vi "Fpga-MicroBlaze_lwIP.vi"() -> ()   [LabVIEW 2017, in "My Network FPGA v1.lvlib"]
uses:
  Example SubVIs/My Network FPGA v1.lvlib
  <instrlib>/_niInstr/Streaming/v1/Common/Stream State.ctl
  <vilib>/Platform/TimedLoop/XDataNode/timing_clust.ctl
  <vilib>/Platform/TimedLoop/XDataNode/nitl_modes.ctl
  <vilib>/Platform/TimedLoop/XDataNode/wakeup.ctl
  <instrlib>/_niInstr/Network/Ethernet/MAC/CLIP/v1/Resources.ctl
  Example SubVIs/TX Controls.ctl
  <instrlib>/_niInstr/Network/Ethernet/MAC/CLIP/v1/niInstr Ethernet MAC - CLIP v1.lvclass
  C:/Program Files (x86)/National Instruments/LabVIEW 2017/instr.lib/_niInstr/Network/Ethernet/MAC/API/v1/FPGA/niInstr Ethernet MAC v1.lvclass
  <instrlib>/_niInstr/Network/API/v1/FPGA/Address Space/niInstr Network API FPGA Address Space v1.lvclass
  C:/Program Files (x86)/National Instruments/LabVIEW 2017/instr.lib/_niInstr/Instruction Framework/v1/FPGA/Interfaces/Address Space Collection/Address Space Collection.lvclass
  <instrlib>/_niInstr/FIFO Register Bus/v1/FPGA/niInstr FIFO Register Bus v1 FPGA.lvclass
  C:/Program Files (x86)/National Instruments/LabVIEW 2017/instr.lib/_niInstr/Instruction Framework/v1/FPGA/Interfaces/Instruction Producer/Instruction Producer.lvclass
  <vilib>/rvi/Emulation/niFpgaSctlEmulationGetInTimedLoop.vi
  <vilib>/rvi/Emulation/niFpgaEmulationReportErrorSimple.vi
  <vilib>/rvi/Emulation/niFpgaGetClockAttributes.vi
  <vilib>/rvi/Emulation/niFpgaCriticalErrorInLSC.vi
  <vilib>/rvi/eio/common/nirviEmuTemplateMethod_errors.vi
  <vilib>/rvi/interface/RandomDataEmulation/niFpgaRandomDataHandleErrors.vi
  <vilib>/Platform/TimedLoop/XDataNode/XDataNode.xnode
  <vilib>/eio/EIONode/EIONode.xnode
  <vilib>/rvi/DataTransferAndStorage/Container/XNode/niFpgaContainer.xnode
  <vilib>/rvi/interface/RandomDataEmulation/nirviRandomDataFpgaReadWriteTemplate.vi
  <vilib>/Platform/TimedLoop/XDataNode/XDNodeRunTimeDep.lvlib
  <instrlib>/_niInstr/Instruction Framework/v1/FPGA/Top Level Bus/Register Configuration/Register Configuration.lvclass
  <instrlib>/_niInstr/Network/API/v1/FPGA/niInstr Network API FPGA v1.lvclass
  <instrlib>/_niInstr/Streaming/v1/Common/niInstr Streaming v1 Common.lvlib
panel:
  out "AXI_STR_RXD_tready 1":bool
  out "tvalid 1":bool
  out "tdata 1":u32
  out "tlast 1":bool
  out "AXI_STR_RXD_tready_Count 1":u16
  out "tvalid_Count 1":u16
  out "tlast_Count 1":u16
  out "tdata_LastNonZero 1":u32
  out "AXI_STR_RXD_tready 2":bool
  out "tvalid 2":bool
  out "tdata 2":u32
  out "tlast 2":bool
  out "AXI_STR_RXD_tready_Count 2":u16
  out "tvalid_Count 2":u16
  out "tlast_Count 2":u16
  out "tdata_LastNonZero 2":u32
  in  "GPIO #1 in":u32
  out "GPIO #1 out":u32
  in  "GPIO #2 in":u32
  out "GPIO #2 out":u32
  in  "Interrupt #0":bool
  in  "Interrupt #1":bool
  in  "Tab Control":T1(tab)
  in  "UDP Source Port 0":u16=43981
  in  "UDP Destination Port 0":u16=61185
  in  "preferred datagram size 0":u16=1472
  in  "Port 0 RX/TX":enum32{"RX", "TX"}(tab)
  in  "Port 0 RX Clear Counts":bool
  out "Port 0 RX Good Frames Count":u32
  out "Port 0 RX Error Frames Count":u32
  out "Port 0 RX Received Columns Count":u32
  out "Port 0 RX Dropped Columns Count":u32
  out "Port 0 RX Data":u64 format="%.0x"
  in  "stream.num samples 0":u64
  in  "stream.request state 0":T2
  out "stream.metadata 0":u64
  out "stream.samples transferred 0":u64
  out "stream.state 0":T2
  in  "Port 1 RX/TX":enum32{"RX", "TX"}(tab)
  in  "Use Pattern Gen":bool
  in  "max frame payload":u16=1472
  in  "minimum packet interval":u32=1
  out "mgtrefclks_locked":bool
  out "mgtrefclks_valid":bool
  out "posc_complete":bool
  out "aBlockLockPort0":bool
  out "aBlockLockPort1":bool
  out "sPort0_Power_Good":bool
  out "sPort1_Power_Good":bool
  out "signal_detect_Port0":bool
  out "signal_detect_Port1":bool
  in  "fifo reg bus ctrl 0":u32
  out "fifo reg bus status 0":u32
  out "fifo reg bus data 0":u64
  # "License Note\n\nThis example makes use of code under the LGPLv2 license in the Socketed CLIP to support 10 Gigabit Ethernet.  You may find the source and build instructions for this component in the CLIP directory."
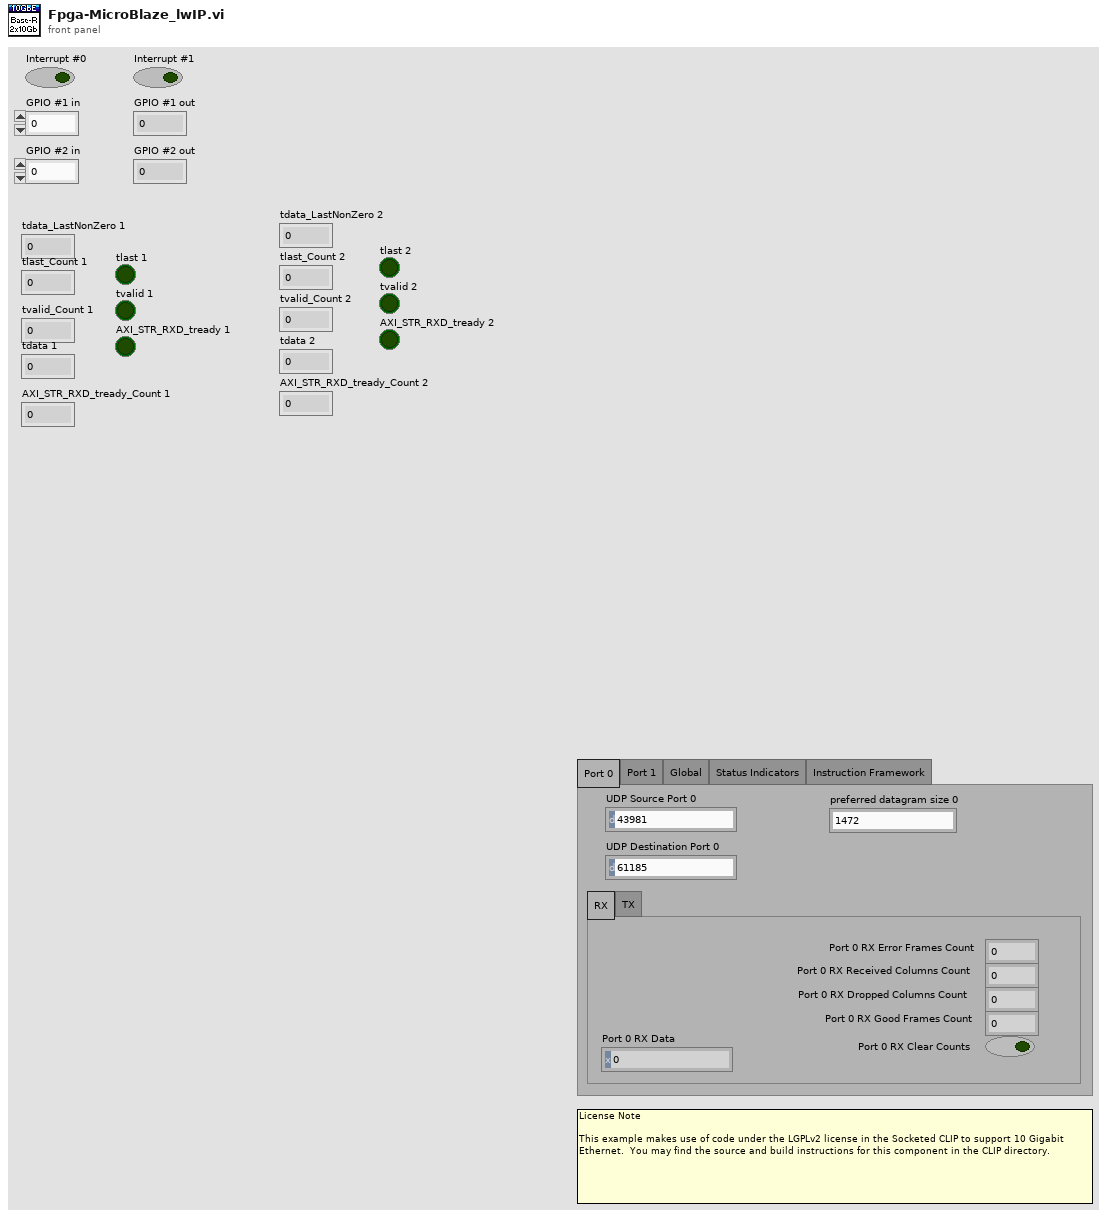
[diagram p1: front panel]
types:
  T1 = enum32{"Port 0", "Port 1", "Global", "Status Indicators", "Instruction Framework"}
  T2 = typedef "niInstr Streaming v1 Common.lvlib/Stream State.ctl" = enum8{"Idle", "Finite Transfer", "Continuous", "Done", "Error", "Not Ready", "Cancel"}
  T3 = typedef "niInstr Ethernet MAC - CLIP v1.lvclass/Resources.ctl" = cluster{"RX":cluster{"TData":refnum<k21>, "TValid":refnum<k21>, "TKeep":refnum<k21>, "TLast":refnum<k21>, "TUser":refnum<k21>}, "TX":cluster{"TData":refnum<k21>, "TValid":refnum<k21>, "TKeep":refnum<k21>, "TLast":refnum<k21>, "TReady":refnum<k21>}, "Pause resources":cluster{"cPauseValuePort":refnum<k21>, "cPauseReqPort":refnum<k21>}, "MAC Clock":refnum<k21>}
  T4 = typedef "XDNodeRunTimeDep.lvlib/timing_clust.ctl" = cluster{"Expected End [f-1]":u64, "Actual End [f-1]":u64, "Finished Late? [f-1]":bool, "Expected End [i-1]":u64, "Actual End [i-1]":u64, "Finished Late? [i-1]":bool, "Expected Start [i]":u64, "Actual Start [i]":u64, "Expected Start [f]":u64, "Actual Start [f]":u64, "Source Name":string, "Structure Name":string, "Period":i64, "Deadline":i64, "Offset":i64, "Start":i64, "Priority":i32, "Timeout":i32, "Mode":T5, "Wakeup Reason":T6, "Error":errorcluster, "Source Type":string, "Secondary Source Type":string, "Global End Time":u64, "Global Start Time":u64, "Frame Duration":u64, "Iteration Duration":u64, "Assigned CPU":i32, "I/O Scan Engine Mode":u32}
  T5 = typedef "XDNodeRunTimeDep.lvlib/nitl_modes.ctl" = enum32{"No Change", "Process missed periods, maintain original phase", "Discard missed periods, maintain original phase", "Process missed periods, ignore original phase", "Discard missed periods, ignore original phase"}
  T6 = typedef "XDNodeRunTimeDep.lvlib/wakeup.ctl" = enum32{"Normal", "Aborted", "Asynchronous wakeup", "Timing source error", "Timed loop error", "Timeout"}
  T7 = typedef "My Network FPGA v1.lvlib/TX Controls.ctl" = cluster{"UDP Source Port":u16, "UDP Destination Port":u16, "preferred datagram size":u16, "Use Pattern Gen":bool, "max frame payload":u16, "minimum packet interval":u32, "stream.num samples 0":u64, "stream.request state 0":T2}
  T8 = cluster{"Port RX Good Frames Count":u32, "Port RX Received Columns Count":u32, "Port RX Dropped Columns Count":u32, "Port RX Error Frames Count":u32, "Port RX Data":u64}
  T9 = typedef "My Network FPGA v1.lvlib/TX Indicators.ctl" = cluster{"stream.state 0":T2, "stream.metadata 0":u64, "stream.samples transferred 0":u64}
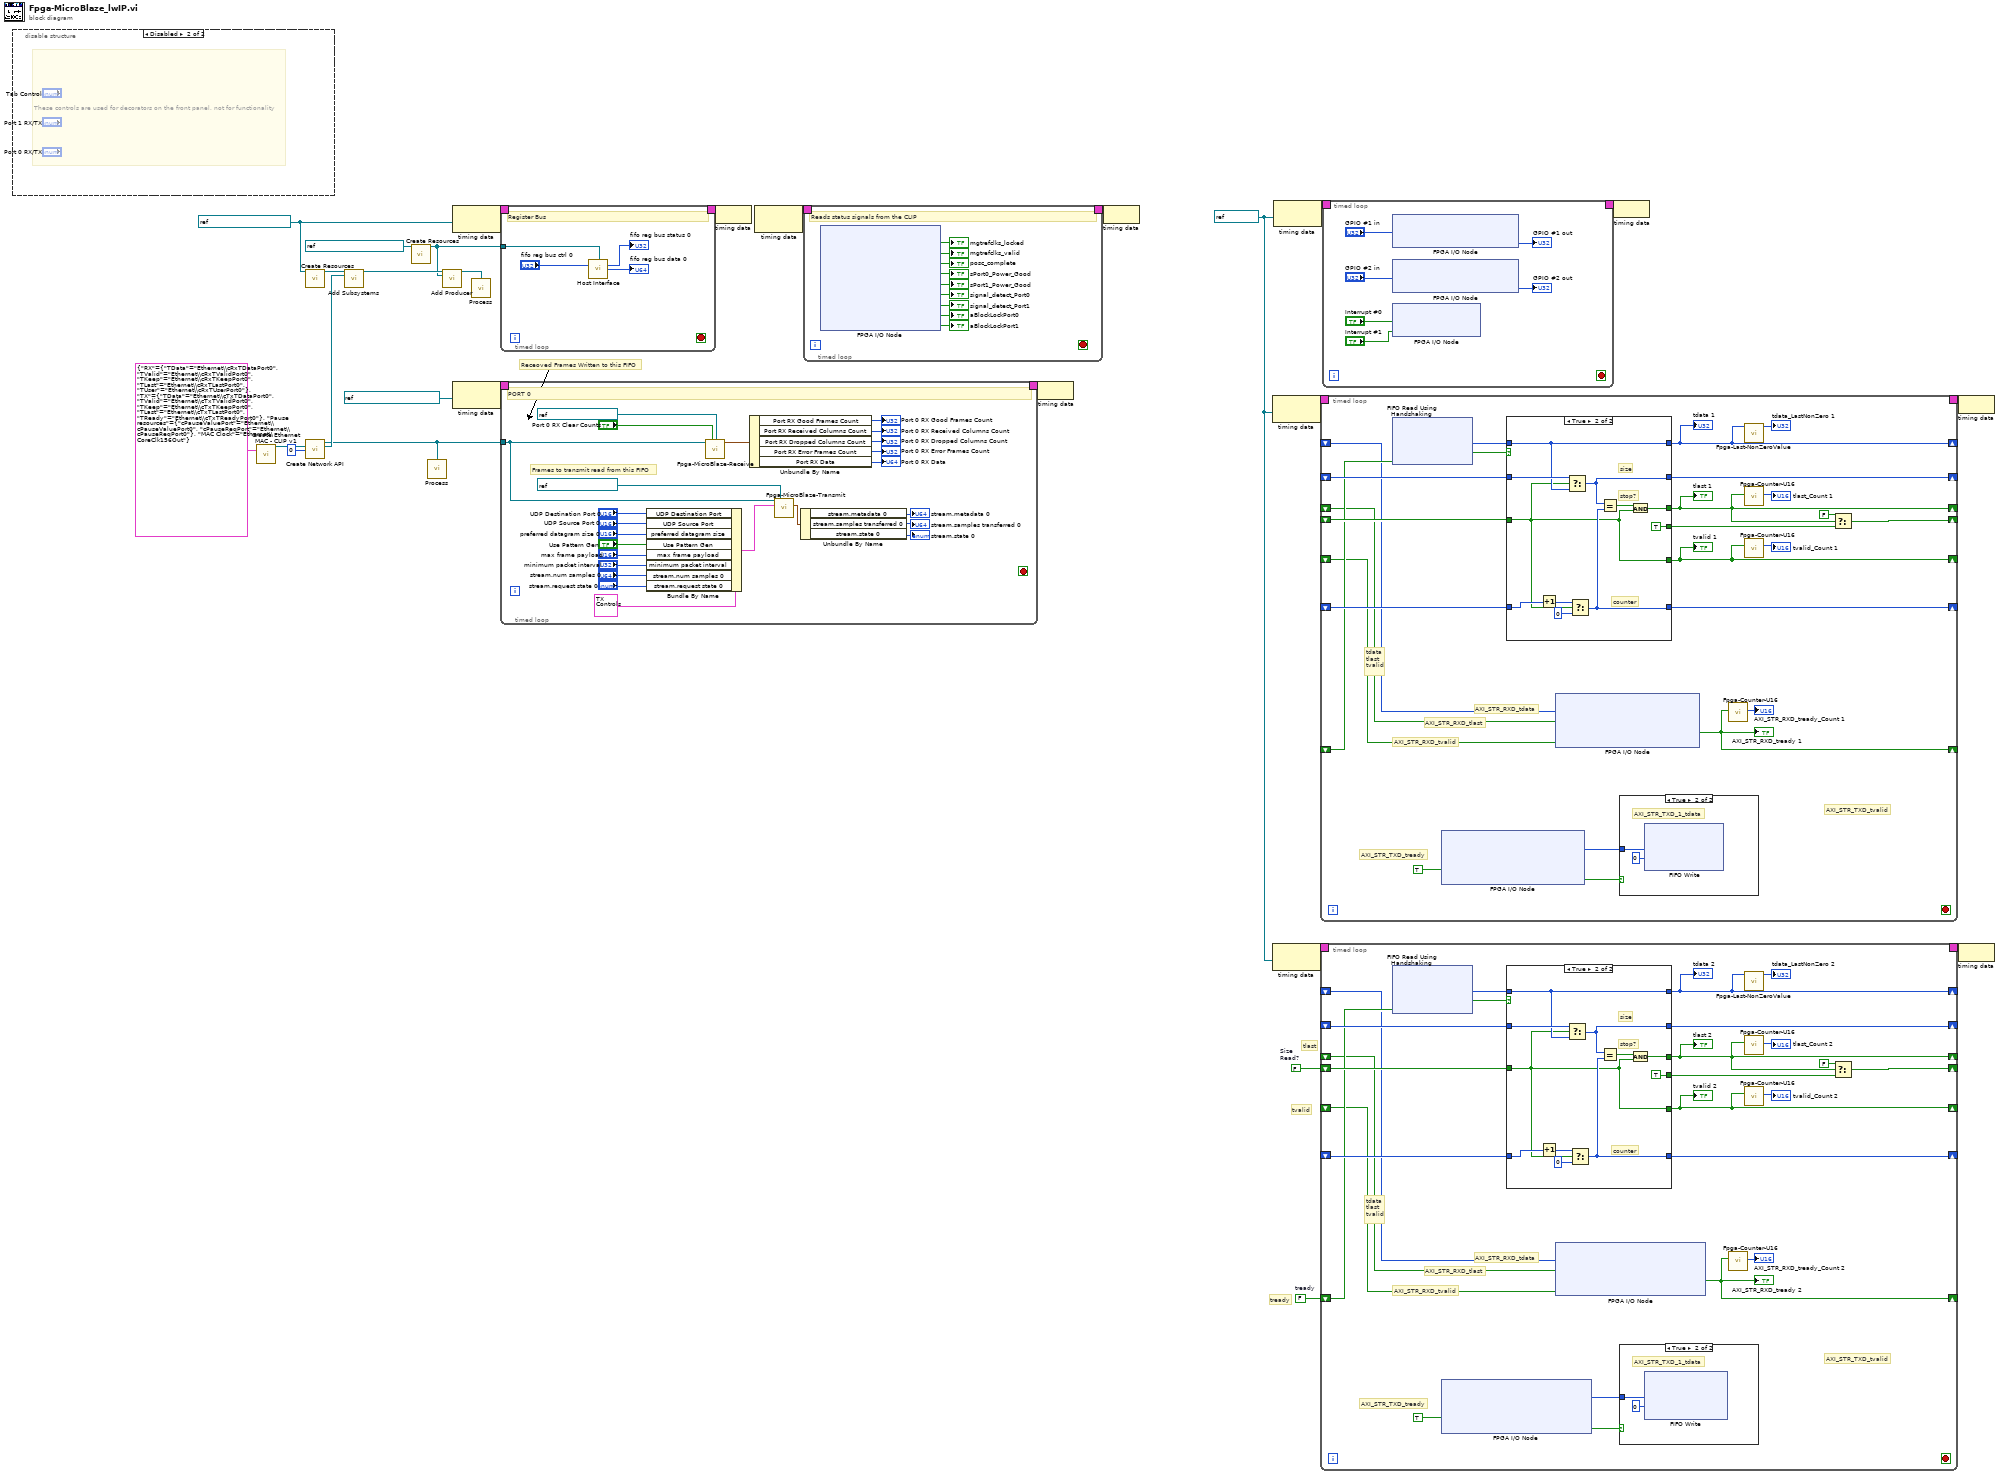
[diagram p0: block diagram]
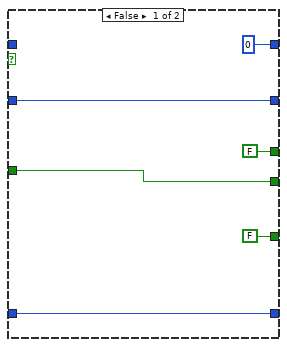
[diagram p3: hidden frame]
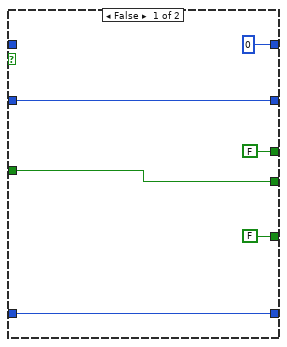
[diagram p5: hidden frame]
diagram:
  w2 = FALSE  # Size Read?
  w3 = FALSE  # tready
  w1 = refnum<k21> "100MHz" ("Source Name")
  w22 = refnum<k21> "40 MHz Onboard Clock" ("Source Name")
  # "tlast"
  # "tvalid"
  # "tready"
  # "Receoved Frames Written to this FIFO"
  n1 = disable-structure shown="Disabled" {
    frame Enabled {
    }
    frame Disabled {
      # "These controls are used for decorators on the front panel, not for functionality"
    }
  }
  n2 = call <instrlib>:"Create Ethernet MAC - CLIP v1.vi"("Ethernet AXI4-S Resources"=T3 {"RX"={"TData"="Ethernet\\cRxTDataPort0", "TValid"="Ethernet\\cRxTValidPort0", "TKeep"="Ethernet\\cRxTKeepPort0", "TLast"="Ethernet\\cRxTLastPort0", "TUser"="Ethernet\\cRxTUserPort0"}, "TX"={"TData"="Ethernet\\cTxTDataPort0", "TValid"="Ethernet\\cTxTValidPort0", "TKeep"="Ethernet\\cTxTKeepPort0", "TLast"="Ethernet\\cTxTLastPort0", "TReady"="Ethernet\\cTxTReadyPort0"}, "Pause resources"={"cPauseValuePort"="Ethernet\\cPauseValuePort0", "cPauseReqPort"="Ethernet\\cPauseReqPort0"}, "MAC Clock"="Ethernet\\CoreClk156Out"}) -> ("niInstr Ethernet MAC - CLIP v1.lvclass out"=w18:refnum<class "niInstr Ethernet MAC - CLIP v1.lvclass">)  [unwired: 14 in]
  n3 = call <instrlib>:"Create Resources.vi"("register clock"=w22) -> ("register configuration"=w17:refnum<class "Register Configuration.lvclass">)  [unwired: 14 in]
  n4 = call <instrlib>:"Create Network API.vi"("niInstr Ethernet MAC v1.lvclass"=w18, "instance"=u8 0 ("Instance")) -> ("niInstr Network API FPGA v1.lvclass"=w11:refnum<class "niInstr Network API FPGA v1.lvclass">, "Address Space Collection"=w16:refnum<class "niInstr Network API FPGA Address Space v1.lvclass">)  [unwired: 12 in]
  n5 = call <instrlib>:"Add Subsystems.vi"("register configuration in"=w17, "subsystems"=w16) -> ("register configuration out"=w15:refnum<class "Register Configuration.lvclass">)  [unwired: 13 in]
  n6 = call <instrlib>:"Create Resources.vi"("instruction fifo"=refnum<k21> "reg.host instruction fifo 0" ("FIFO")) -> ("fifo register bus"=w10:refnum<class "niInstr FIFO Register Bus v1 FPGA.lvclass">)  [unwired: 14 in]
  n7 = call <instrlib>:"Process.vi"("niInstr Network API FPGA v1.lvclass"=w11) -> ()  [unwired: 15 in]
  n8 = call <instrlib>:"Add Producer.vi"("register configuration in"=w15, "instruction producer"=w10) -> ("register configuration out"=w21:refnum<class "Register Configuration.lvclass">)  [unwired: 13 in]
  n9 = node-c288(w22) -> (w25:T4)
  n10 = node-c288(refnum<k21> "Ethernet\\CoreClk156Out" ("Source Name")) -> (w20:T4)
  n11 = call <instrlib>:"Process.vi"("register configuration"=w21) -> ()  [unwired: 15 in]
  n12 = timed-loop {
    timing: w25 -> [_]
    timing-out: [_] -> w24
    tunnel: w10 -> [w31]
    stop <- _ stop-if-true
    # "Register Bus"
    n13 = call <instrlib>:"Host Interface.vi"("fifo register bus"=w31, "fifo reg bus ctrl 0"="fifo reg bus ctrl 0") -> ("fifo reg bus status 0"=→"fifo reg bus status 0":u32, "fifo reg bus data 0"=→"fifo reg bus data 0":u64)  [unwired: 12 in]
  }
  n14 = timed-loop {
    timing: w20 -> [_]
    timing-out: [_] -> w19
    tunnel: w11 -> [w49]
    stop <- _ stop-if-true
    # "Frames to transmit read from this FIFO"
    # "PORT 0"
    n15 = Bundle By Name(cluster=T7 {"UDP Source Port"=43981, "UDP Destination Port"=61185, "preferred datagram size"=1400, "Use Pattern Gen"=FALSE, "max frame payload"=1472, "minimum packet interval"=1, "stream.num samples 0"=0, "stream.request state 0"=enum."Idle"} ("Controls"), "UDP Destination Port"="UDP Destination Port 0", "UDP Source Port"="UDP Source Port 0", "preferred datagram size"="preferred datagram size 0", "Use Pattern Gen"="Use Pattern Gen", "max frame payload"="max frame payload", "minimum packet interval"="minimum packet interval", "stream.num samples 0"="stream.num samples 0", "stream.request state 0"="stream.request state 0") -> (w47:T7)
    n16 = call "Fpga-MicroBlaze-Receive.vi"("niInstr Network API FPGA v1.lvclass"=w49, "Port RX Clear Counts"="Port 0 RX Clear Counts", "RX FIFO"=refnum<k21> "Port 0 Host RX FIFO" ("Host RX FIFO")) -> ("debug data"=w56:T8)  [unwired: 12 in]
    n17 = Unbundle By Name(w56) -> ("Port RX Good Frames Count"=→"Port 0 RX Good Frames Count":u32, "Port RX Received Columns Count"=→"Port 0 RX Received Columns Count":u32, "Port RX Dropped Columns Count"=→"Port 0 RX Dropped Columns Count":u32, "Port RX Error Frames Count"=→"Port 0 RX Error Frames Count":u32, "Port RX Data"=→"Port 0 RX Data":u64)
    n18 = call "Fpga-MicroBlaze-Transmit.vi"("Network API"=w49, "FIFO In"=refnum<k21> "Port 0 Host TX FIFO", "Controls"=w47) -> ("Indicators"=w39:T9)  [unwired: 12 in]
    n19 = Unbundle By Name(w39) -> ("stream.metadata 0"=→"stream.metadata 0":u64, "stream.samples transferred 0"=→"stream.samples transferred 0":u64, "stream.state 0"=→"stream.state 0":T2)
  }
  n20 = node-c288(w24) -> ()
  n21 = node-c288() -> (w27:T4)  [unwired: 1 in]
  n22 = timed-loop {
    timing: w27 -> [_]
    timing-out: [_] -> w26
    stop <- _ stop-if-true
    # "Reads status signals from the CLIP"
    n23 = xnode "FPGA I/O Node"() -> ("Ethernet\\MgtRefClks_Locked"=→"mgtrefclks_locked":bool, "Ethernet\\MgtRefClks_Valid"=→"mgtrefclks_valid":bool, "Ethernet\\POSC_Complete"=→"posc_complete":bool, "Ethernet\\sPort0_Power_Good"=→"sPort0_Power_Good":bool, "Ethernet\\sPort1_Power_Good"=→"sPort1_Power_Good":bool, "Ethernet\\signal_detect_Port0"=→"signal_detect_Port0":bool, "Ethernet\\signal_detect_Port1"=→"signal_detect_Port1":bool, "Ethernet\\aBlockLockPort0"=→"aBlockLockPort0":bool, "Ethernet\\aBlockLockPort1"=→"aBlockLockPort1":bool)  [unwired: 9 in, 9 out]
  }
  n24 = node-c288(w19) -> ()
  n25 = node-c288(w26) -> ()
  n26 = node-c288(w1) -> (w5:T4)
  n27 = node-c288(w1) -> (w7:T4)
  n28 = node-c288(w1) -> (w9:T4)
  n29 = timed-loop {
    timing: w5 -> [_]
    timing-out: [_] -> w4
    shift-right: [w76] -> _
    shift-left: _ -> [w94]
    shift-right: [w91] -> _
    shift-left: _ -> [w93]
    shift-right: [w89] -> _
    shift-left: _ -> [w90]
    shift-right: [w72] -> _
    shift-left: _ -> [w82]
    shift-right: [w71] -> _
    shift-left: _ -> [w88]
    shift-right: [w86] -> _
    shift-left: _ -> [w84]
    shift-right: [w75] -> _
    shift-left: _ -> [w83]
    stop <- _ stop-if-true
    # "AXI_STR_TXD_tvalid"
    # "AXI_STR_TXD_tready"
    # "AXI_STR_RXD_tvalid"
    # "AXI_STR_RXD_tlast"
    # "AXI_STR_RXD_tdata"
    # "tdata\ntlast\ntvalid"
    n30 = xnode ("FIFO Read Using Handshaking")("Ready for Output"=w88) -> ("Element"=w92:u32, "Output Valid"=w95:bool)  [unwired: 1 in, 1 out]
    n31 = xnode "FPGA I/O Node"("d_microblaze_i\\AXI_STR_TXD_tready"=TRUE ("d_microblaze\\AXI_STR_TXD_tready")) -> ("d_microblaze_i\\AXI_STR_TXD_tdata"=w79:u32, "d_microblaze_i\\AXI_STR_TXD_tvalid"=w80:bool)  [unwired: 4 in, 5 out]
    n32 = case shown="True" w95 {
      tunnel: w94 -> [w102 w104]
      tunnel: [w102 TRUE ("Size\nRead?")] -> w77
      tunnel: w93 -> [w103 w114]
      tunnel: w92 -> [_ w109]
      tunnel: [w103 w108] -> w91
      tunnel: w90 -> [w101 w113]
      tunnel: [w101 w107] -> w89
      tunnel: [FALSE ("Size\nRead?") w104] -> w72
      tunnel: [u32 0 ("Element") w109] -> w86
      tunnel: [FALSE w105] -> w75
      frame False {
      }
      frame True {
        # "stop?"
        # "size"
        # "counter"
        n33 = Increment(x=w113) -> (x+1=w111:u32)
        n34 = Select(t=w114, s=w104, f=w109) -> (s? t:f=w108:u32)
        n35 = Select(t=w111, s=w104, f=u32 0) -> (s? t:f=w107:u32)
        n36 = Equal?(x=w108, y=w107) -> (x = y?=w106:bool)
        n37 = And(x=w106, y=w104) -> (x .and. y?=w105:bool)
      }
    }
    "tvalid 1" <- w72
    "tdata 1" <- w86
    "tlast 1" <- w75
    n38 = xnode "FPGA I/O Node"("d_microblaze_i\\AXI_STR_RXD_tdata"=w84, "d_microblaze_i\\AXI_STR_RXD_tlast"=w83, "d_microblaze_i\\AXI_STR_RXD_tvalid"=w82) -> ("d_microblaze_i\\AXI_STR_RXD_tready"=w71:bool)  [unwired: 4 in, 4 out]
    "AXI_STR_RXD_tready 1" <- w71
    n39 = case shown="True" w80 {
      tunnel: w79 -> [_ w97]
      frame False {
      }
      frame True {
        # "AXI_STR_TXD_1_tdata"
        n40 = xnode ("FIFO Write")("Element"=w97, "Timeout"=0) -> ()  [unwired: 1 in, 2 out]
      }
    }
    n41 = call "Fpga-Counter-U16.vi"("d_mcs_i\\IO_BUS_read_strobe"=w71) -> ("Numeric"=→"AXI_STR_RXD_tready_Count 1":u16)  [unwired: 10 in]
    n42 = call "Fpga-Last-NonZeroValue.vi"("d_mcs_i\\IO_BUS_write_data in"=w86) -> ("d_mcs_i\\IO_BUS_write_data out"=→"tdata_LastNonZero 1":u32)  [unwired: 10 in]
    n43 = call "Fpga-Counter-U16.vi"("d_mcs_i\\IO_BUS_read_strobe"=w75) -> ("Numeric"=→"tlast_Count 1":u16)  [unwired: 10 in]
    n44 = call "Fpga-Counter-U16.vi"("d_mcs_i\\IO_BUS_read_strobe"=w72) -> ("Numeric"=→"tvalid_Count 1":u16)  [unwired: 10 in]
    n45 = Select(t=FALSE, s=w75, f=w77) -> (s? t:f=w76:bool)
  }
  n46 = timed-loop {
    timing: w7 -> [_]
    timing-out: [_] -> w6
    shift-right: [w122] -> _
    shift-left: w2 -> [w140]
    shift-right: [w137] -> _
    shift-left: _ -> [w139]
    shift-right: [w135] -> _
    shift-left: _ -> [w136]
    shift-right: [w118] -> _
    shift-left: _ -> [w128]
    shift-right: [w117] -> _
    shift-left: w3 -> [w134]
    shift-right: [w132] -> _
    shift-left: _ -> [w130]
    shift-right: [w121] -> _
    shift-left: _ -> [w129]
    stop <- _ stop-if-true
    # "AXI_STR_TXD_tvalid"
    # "AXI_STR_TXD_tready"
    # "AXI_STR_RXD_tvalid"
    # "AXI_STR_RXD_tlast"
    # "AXI_STR_RXD_tdata"
    # "tdata\ntlast\ntvalid"
    n47 = xnode ("FIFO Read Using Handshaking")("Ready for Output"=w134) -> ("Element"=w138:u64, "Output Valid"=w141:bool)  [unwired: 1 in, 1 out]
    n48 = xnode "FPGA I/O Node"("d_microblaze_i\\AXI_STR_TXD_1_tready"=TRUE ("d_microblaze\\AXI_STR_TXD_tready")) -> ("d_microblaze_i\\AXI_STR_TXD_1_tdata"=w125:u32, "d_microblaze_i\\AXI_STR_TXD_1_tvalid"=w126:bool)  [unwired: 4 in, 5 out]
    n49 = case shown="True" w141 {
      tunnel: w140 -> [w148 w150]
      tunnel: [w148 TRUE ("Size\nRead?")] -> w123
      tunnel: w139 -> [w149 w160]
      tunnel: w138 -> [_ w155]
      tunnel: [w149 w154] -> w137
      tunnel: w136 -> [w147 w159]
      tunnel: [w147 w153] -> w135
      tunnel: [FALSE ("Size\nRead?") w150] -> w118
      tunnel: [u32 0 ("Element") w155] -> w132
      tunnel: [FALSE w151] -> w121
      frame False {
      }
      frame True {
        # "stop?"
        # "size"
        # "counter"
        n50 = Increment(x=w159) -> (x+1=w157:u32)
        n51 = Select(t=w160, s=w150, f=w155) -> (s? t:f=w154:u64)
        n52 = Select(t=w157, s=w150, f=u32 0) -> (s? t:f=w153:u32)
        n53 = Equal?(x=w154, y=w153) -> (x = y?=w152:bool)
        n54 = And(x=w152, y=w150) -> (x .and. y?=w151:bool)
      }
    }
    "tvalid 2" <- w118
    "tdata 2" <- w132
    "tlast 2" <- w121
    n55 = xnode "FPGA I/O Node"("d_microblaze_i\\AXI_STR_RXD_1_tdata"=w130, "d_microblaze_i\\AXI_STR_RXD_1_tlast"=w129, "d_microblaze_i\\AXI_STR_RXD_1_tvalid"=w128) -> ("d_microblaze_i\\AXI_STR_RXD_1_tready"=w117:bool)  [unwired: 4 in, 4 out]
    "AXI_STR_RXD_tready 2" <- w117
    n56 = case shown="True" w126 {
      tunnel: w125 -> [_ w143]
      frame False {
      }
      frame True {
        # "AXI_STR_TXD_1_tdata"
        n57 = xnode ("FIFO Write")("Element"=w143, "Timeout"=0) -> ()  [unwired: 1 in, 2 out]
      }
    }
    n58 = call "Fpga-Counter-U16.vi"("d_mcs_i\\IO_BUS_read_strobe"=w117) -> ("Numeric"=→"AXI_STR_RXD_tready_Count 2":u16)  [unwired: 10 in]
    n59 = call "Fpga-Last-NonZeroValue.vi"("d_mcs_i\\IO_BUS_write_data in"=w132) -> ("d_mcs_i\\IO_BUS_write_data out"=→"tdata_LastNonZero 2":u32)  [unwired: 10 in]
    n60 = call "Fpga-Counter-U16.vi"("d_mcs_i\\IO_BUS_read_strobe"=w121) -> ("Numeric"=→"tlast_Count 2":u16)  [unwired: 10 in]
    n61 = call "Fpga-Counter-U16.vi"("d_mcs_i\\IO_BUS_read_strobe"=w118) -> ("Numeric"=→"tvalid_Count 2":u16)  [unwired: 10 in]
    n62 = Select(t=FALSE, s=w121, f=w123) -> (s? t:f=w122:bool)
  }
  n63 = timed-loop {
    timing: w9 -> [_]
    timing-out: [_] -> w8
    stop <- _ stop-if-true
    n64 = xnode "FPGA I/O Node"("d_microblaze_i\\gpio_rtl_tri_i"="GPIO #1 in") -> ("d_microblaze_i\\gpio_rtl_0_tri_o"=→"GPIO #1 out":u32)  [unwired: 2 in, 2 out]
    n65 = xnode "FPGA I/O Node"("d_microblaze_i\\gpio_rtl_1_tri_i"="GPIO #2 in") -> ("d_microblaze_i\\gpio_rtl_2_tri_o"=→"GPIO #2 out":u32)  [unwired: 2 in, 2 out]
    n66 = xnode "FPGA I/O Node"("d_microblaze_i\\In0"="Interrupt #0", "d_microblaze_i\\In1"="Interrupt #1") -> ()  [unwired: 2 in, 2 out]
  }
  n67 = node-c288(w8) -> ()
  n68 = node-c288(w4) -> ()
  n69 = node-c288(w6) -> ()
